vi "stop.vi"(8 "error in (no error)":errorcluster, 11 "Analog_Output in":refnum<class "Analog_Output.lvclass">) -> (0 "error out":errorcluster, 3 "Analog_Output out":refnum<class "Analog_Output.lvclass">)   [LabVIEW 2013, in "Analog_Output.lvclass"]
uses:
  Analog_Output.lvclass
  Analog_Output.lvclass/Analog_Output.ctl
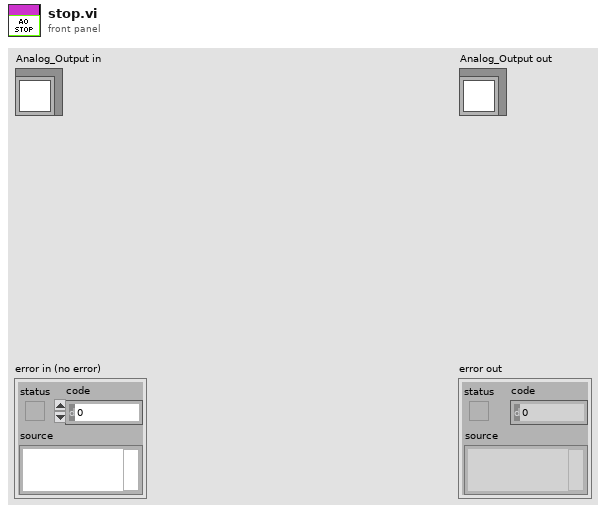
[diagram p1: front panel]
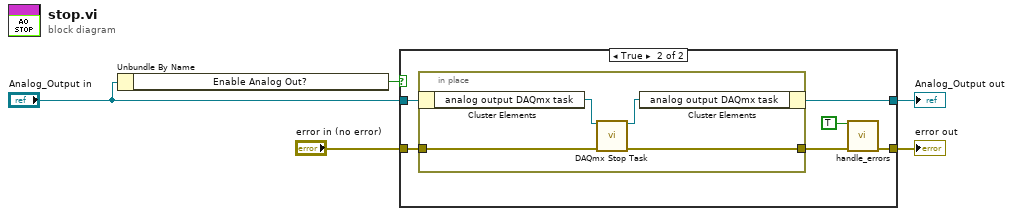
[diagram p0: block diagram]
diagram:
  n1 = Unbundle By Name("Analog_Output in") -> ("Enable Analog Out?"=w3:bool)
  n2 = case shown="True" w3 {
    tunnel: [w7 w11] -> w4
    tunnel: "error in (no error)" -> [w7 w13]
    tunnel: "Analog_Output in" -> [w6 w9]
    tunnel: [w6 w8] -> w1
    frame False {
    }
    frame True {
      n3 = in-place {
        in-place-border: w13 -> [w17]
        in-place-border: [w16] -> w12
        n4 = in-place-cluster #1(w9) -> ("analog output DAQmx task"=w14:refnum<k21>)
        n5 = call <vilib>:"DAQmx Stop Task.vi"("task/channels in"=w14, "error in"=w17) -> ("task out"=w15:refnum<k21>, "error out"=w16:errorcluster)  [unwired: 12 in]
        n6 = in-place-cluster #1("analog output DAQmx task"=w15) -> (w8:refnum<class "Analog_Output.lvclass">)
      }
      n7 = call "handle_errors.vi"("Exit Operation"=TRUE ("Exit Measurement"), "error in (no error)"=w12) -> ("error out"=w11:errorcluster)  [unwired: 13 in]
    }
  }
  "error out" <- w4
  "Analog_Output out" <- w1
